vi "Msg to Send.vi"(9 "Alias":string, 10 "Nest Actor":refnum<class "LVCAM.lvclass">) -> (3 "Create Msg out":refnum<class "Create Msg.lvclass">)   [LabVIEW 2021, in "Create.lvlib" / "Create Msg.lvclass"]
uses:
  Create Msg.lvclass
  AAM/LVCAM/LVCAM.lvclass
  Create Msg.lvclass/Create Msg.ctl
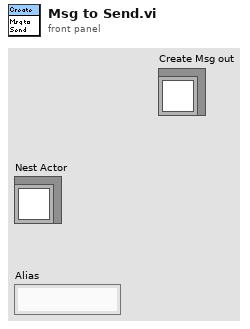
[diagram p1: front panel]
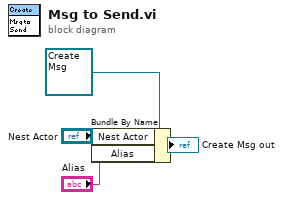
[diagram p0: block diagram]
diagram:
  n1 = Bundle By Name(cluster=refnum<class "Create Msg.lvclass"> refnum ("Create Msg in"), "Nest Actor"="Nest Actor", "Alias"="Alias") -> (→"Create Msg out":refnum<class "Create Msg.lvclass">)
